vi "EditorMethod runListProcess.vi"(5 "currFilePath":path, 7 "state":T4, 8 "error in (no error)":errorcluster, 10 "dataParam":T3, 11 "listboxRefnum":refnum<vi>) -> (0 "error out":errorcluster, 1 "exportData":T1, 2 "newSigInfo":T2, 3 "listboxRefnum out":refnum<vi>)   [LabVIEW 2018]
uses:
  ctl/dataListboxState.ctl
  ctl/editScriptState.ctl
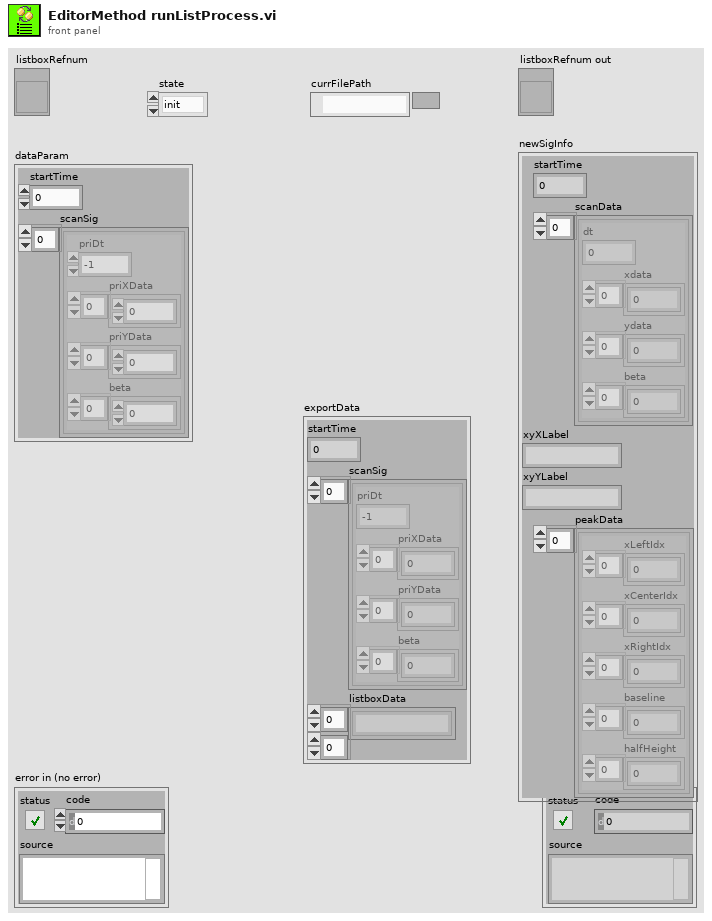
[diagram p1: front panel]
types:
  T1 = cluster{"startTime":dbl, "scanSig":cluster{"priDt":dbl, "priXData":dbl[], "priYData":sgl[], "beta":dbl[]}[], "listboxData":string[][]}
  T2 = cluster{"startTime":dbl, "scanData":cluster{"dt":dbl, "xdata":dbl[], "ydata":sgl[], "beta":dbl[]}[], "xyXLabel":string, "xyYLabel":string, "peakData":cluster{"xLeftIdx":u32[], "xCenterIdx":u32[], "xRightIdx":u32[], "baseline":sgl[], "halfHeight":dbl[]}[]}
  T3 = cluster{"startTime":dbl, "scanSig":cluster{"priDt":dbl, "priXData":dbl[], "priYData":sgl[], "beta":dbl[]}[]}
  T4 = typedef "dataListboxState.ctl" = enum16{"init", "setData", "upd", "getExport"}
  T5 = typedef "editScriptState.ctl" = enum16{"init", "loadScript", "newScript", "runScript", "close"}
  T6 = cluster{"currFilePath":path, "dataParam":cluster{"startTime":dbl, "scanSig":cluster{"priDt":dbl, "priXData":dbl[], "priYData":sgl[], "beta":dbl[]}[]}}
  T7 = cluster{"priDt":dbl, "priXData":dbl[], "priYData":sgl[], "beta":dbl[]}[]
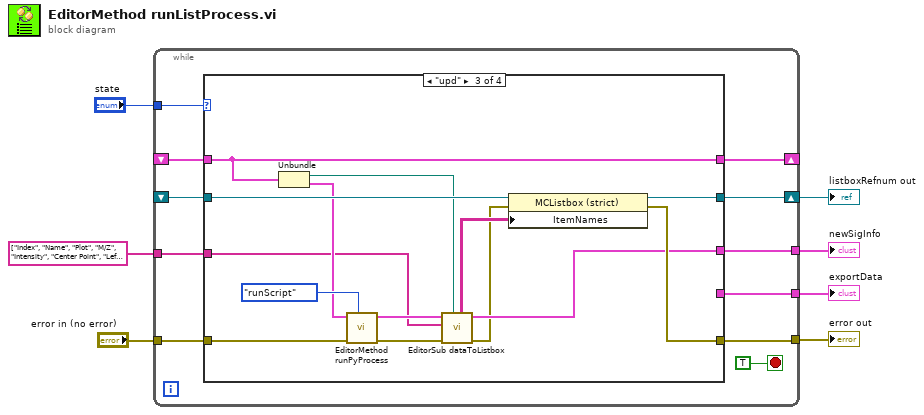
[diagram p0: block diagram]
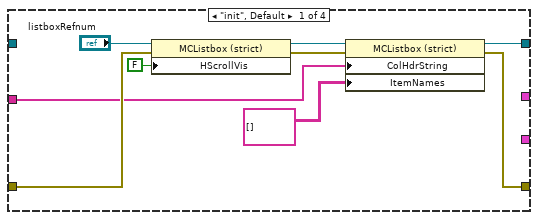
[diagram p2: hidden frame]
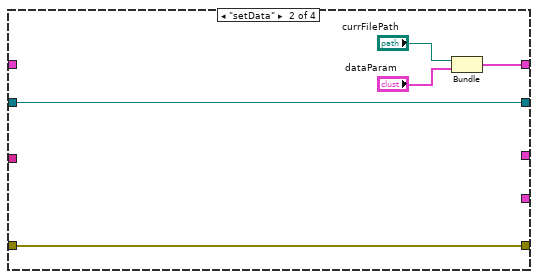
[diagram p3: hidden frame]
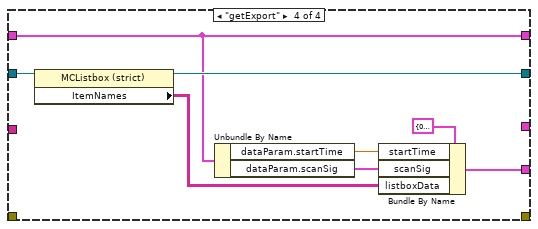
[diagram p4: hidden frame]
diagram:
  n1 = while {
    tunnel: "state" -> [w18]
    shift-right: [w17] -> w2
    shift-left: _ -> [w16]
    tunnel: [w14] -> w6
    tunnel: "error in (no error)" -> [w13]
    tunnel: [w11] -> w4
    shift-right: [w10] -> _
    shift-left: _ -> [w12]
    tunnel: string[] ["Index", "Name", "Plot", "M/Z", "Intensity", "Center Point", "Left Point", "Right Point", "Half Height", "Remark"] ("Column Header Strings[]") -> [w9]
    tunnel: [w8] -> w1
    stop <- TRUE stop-if-true
    n2 = case shown="\"upd\"" w18 {
      tunnel: [w23 w32 w45 w53] -> w17
      tunnel: w16 -> [_ w32 w46 w54]
      tunnel: [w22 w31 w43 _] -> w14
      tunnel: w13 -> [w21 w31 w42 _]
      tunnel: w12 -> [_ _ w41 w50]
      tunnel: [_ _ w37 _] -> w11
      tunnel: [_ w28 w41 w50] -> w10
      tunnel: w9 -> [w20 _ w35 _]
      tunnel: [_ _ _ w49] -> w8
      frame "init", Default {
        n3 = property class="MCListbox (strict)"(reference="listboxRefnum", error in=w21, "HScrollVis"=FALSE ("Visible Items:Horizontal Scrollbar Visible")) -> (reference out=w27:refnum<vi>, error out=w26:errorcluster)
        n4 = property class="MCListbox (strict)"(reference=w27, error in=w26, "ColHdrString"=w20, "ItemNames"=string[][] [] ("Item Names")) -> (reference out=w23:refnum<vi>, error out=w22:errorcluster)
      }
      frame "setData" {
        n5 = Bundle("currFilePath"="currFilePath", "dataParam"="dataParam") -> (w28:T6)  [unwired: 1 in]
      }
      frame "upd" {
        n6 = Unbundle(w41) -> ("currFilePath"=w36:path, "dataParam"=w40:T3)
        n7 = call "EditorMethod runPyProcess.vi"("func"=editScriptState."runScript", "error in (no error)"=w42, "dataParam"=w40) -> ("error out"=w38:errorcluster, "newSigInfo"=w39:T2)  [unwired: 5 in, 2 out]
        n8 = call "EditorSub dataToListbox.vi"("currFilePath"=w36, "error in (no error)"=w38, "listboxColHead"=w35, "newSigInfo in"=w39) -> ("error out"=w33:errorcluster, "newSigInfo out"=w37:T2, "Item Names"=w34:string[][])  [unwired: 5 in]
        n9 = property class="MCListbox (strict)"(reference=w46, error in=w33, "ItemNames"=w34) -> (reference out=w45:refnum<vi>, error out=w43:errorcluster)
      }
      frame "getExport" {
        n10 = property class="MCListbox (strict)"(reference=w54) -> (reference out=w53:refnum<vi>, "ItemNames"=w51:string[][])  [unwired: 1 in, 1 out]
        n11 = Unbundle By Name(w50) -> ("dataParam.startTime"=w48:dbl, "dataParam.scanSig"=w47:T7)
        n12 = Bundle By Name(cluster=T1 {"startTime"=0.0, "scanSig"=[], "listboxData"=[]} ("exportData"), "startTime"=w48, "scanSig"=w47, "listboxData"=w51) -> (w49:T1)
      }
    }
  }
  "error out" <- w6
  "newSigInfo" <- w4
  "listboxRefnum out" <- w2
  "exportData" <- w1
